vi "ConvertTCVolts.vi"(8 "error in (no error)":errorcluster, 10 "T CJC":dbl=25.0, 11 "Vmeas":dbl) -> (0 "error out":errorcluster, 3 "Tmeas":dbl)   [LabVIEW 2014]
uses:
  <vilib>/Analysis/polynomials.llb/Scalar Polynomial Evaluation (DBL).vi
  <vilib>/Analysis/NI_AALPro.lvlib
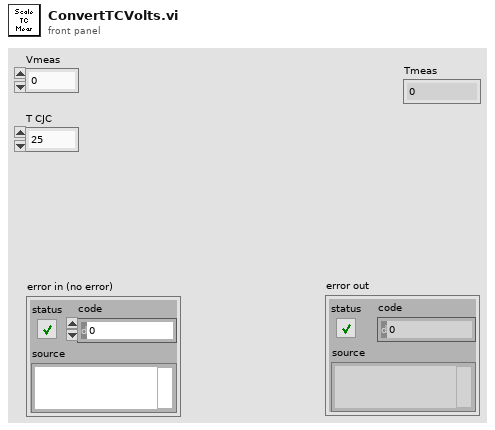
[diagram p1: front panel]
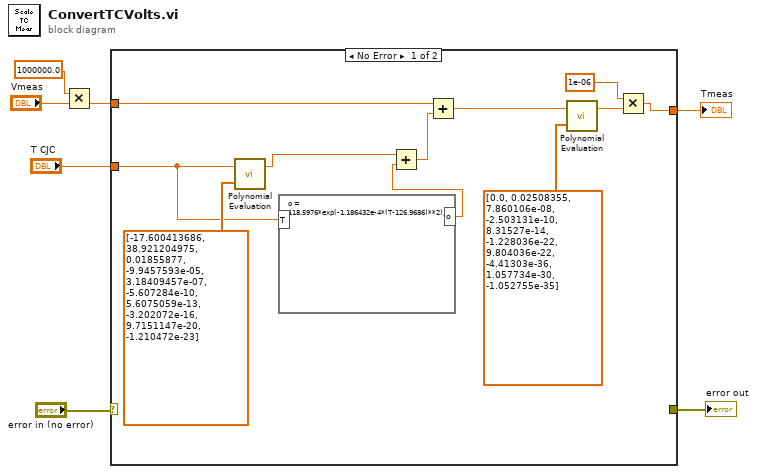
[diagram p0: block diagram]
diagram:
  n1 = Multiply(x=1000000.0, y="Vmeas") -> (x*y=w2:dbl)
  n2 = case shown="No Error" "error in (no error)" {
    selector: "error in (no error)" -> [_ w19]
    tunnel: w2 -> [w17 _]
    tunnel: "T CJC" -> [w14 _]
    tunnel: [w8 _] -> w4
    tunnel: [_ w19] -> w3
    frame No Error {
      n3 = call-poly <vilib>:"Polynomial Evaluation.vi"("P(x)"=dbl[] [-17.600413686, 38.921204975, 0.01855877, -9.9457593e-05, 3.18409457e-07, -5.607284e-10, 5.6075059e-13, -3.202072e-16, 9.7151147e-20, -1.210472e-23], "a"=w14) -> ("P(a)"=w12:dbl)  [unwired: 1 out]
      n4 = formula code="o = 118.5976*exp(-1.186432e-4*(T-126.9686)**2);"("T"=w14) -> ("o"=w13:dbl)
      n5 = Add(x=w12, y=w13) -> (x+y=w11:dbl)
      n6 = Add(x=w17, y=w11) -> (x+y=w16:dbl)
      n7 = call-poly <vilib>:"Polynomial Evaluation.vi"("P(x)"=dbl[] [0.0, 0.02508355, 7.860106e-08, -2.503131e-10, 8.31527e-14, -1.228036e-22, 9.804036e-22, -4.41303e-36, 1.057734e-30, -1.052755e-35], "a"=w16) -> ("P(a)"=w10:dbl)  [unwired: 1 out]
      n8 = Multiply(x=1e-06, y=w10) -> (x*y=w8:dbl)
    }
    frame Error {
    }
  }
  "Tmeas" <- w4
  "error out" <- w3
